vi "DROPBEAR_Model_Updating_Store_Statisitics.vi"(8 "error in (no error)":errorcluster, 11 "DROPBEAR_Model_Updating in":refnum<class "DROPBEAR_Model_Updating.lvclass">) -> (0 "error out":errorcluster, 3 "DROPBEAR_Model_Updating out":refnum<class "DROPBEAR_Model_Updating.lvclass">)   [LabVIEW 2021, in "DROPBEAR_Model_Updating.lvclass"]
uses:
  DROPBEAR_Model_Updating.lvclass
  Online_Statistic/Online_Statistic.lvclass
  Moving_Statistic/Moving_Statistic.lvclass
  Data_Array/Data_Array.lvclass
  DROPBEAR_Model_Updating.lvclass/DROPBEAR_Model_Updating.ctl
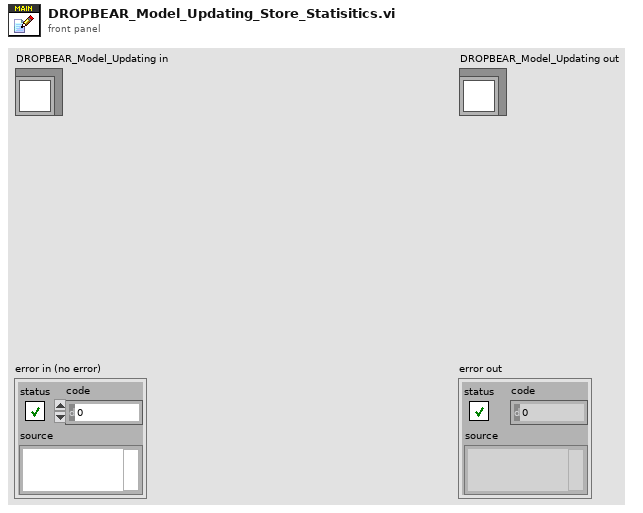
[diagram p1: front panel]
types:
  T1 = cluster{"Data Acquistion Time Cost":refnum<class "Online_Statistic.lvclass">, "FFT Time Cost":refnum<class "Online_Statistic.lvclass">, "Sample Location Time Cost":refnum<class "Online_Statistic.lvclass">, "FEA Time Cost":refnum<class "Online_Statistic.lvclass">, "Frequency Tracking Time Cost":refnum<class "Online_Statistic.lvclass">, "State Tracking Time Cost":refnum<class "Online_Statistic.lvclass">, "Online Cycle Time Cost":refnum<class "Online_Statistic.lvclass">}
  T2 = cluster{"Time Cycle Start":u32, "Time Data Acquire":u32, "Time FFT":u32, "Time KF FFT":u32, "Time Sample":u32, "Time FEA":u32, "Time KF FEA":u32, "Time Cycle End":u32}
  T3 = cluster{"Number_of_samples":i32, "Max":dbl, "Min":dbl, "Cumulative_mean":dbl, "Cumulative_mean_square ":dbl, "Cumulative_variance":dbl}
  T4 = cluster{"Displacement Measured Meters":refnum<class "Moving_Statistic.lvclass">, "Displacement Estimate Meters":refnum<class "Moving_Statistic.lvclass">, "Frequency Measured":refnum<class "Moving_Statistic.lvclass">, "Frequency at Estimate":refnum<class "Moving_Statistic.lvclass">}
  T5 = cluster{"Position Measured Meters":dbl, "Position Measured Nodal":i32, "Position Estimated Meters":dbl, "Position Estimated Nodal":i32, "Frequency Estimated KF":dbl, "Frequency Measured FFT":dbl, "Position Estimated Meters KF":dbl, "Position Estimated Nodal KF":i32, "Mean Cycle time":dbl}
  T6 = cluster{"Modeling Parameters input controls":cluster{"beam_length":dbl, "youngs_modulus":dbl, "torsion_spring":dbl, "beam_height":dbl, "beam_width":dbl, "beam_density":dbl, "number_of_FEA_nodes":i32, "accelerometer_mass":dbl}, "Mockbear input controls":cluster{"Dataset":string, "Resample Method":enum16{"Recorded", "Auto Resample", "Custom Resample"}}, "Simulation Parameters input controls":cluster{"Eigensolver ":enum16{"LabVIEW Cholesky", "LabVIEW General", "LabVIEW Inverse", "LEMP"}, "Models Forcasted":i32, "Max Roller Velocity":dbl, "Max Roller Position Percent":dbl, "Min Roller Position Percent":dbl}, "Program Controls":cluster{"Frequency KF":bool, "Pinned State KF":bool, "FFT Bounding":bool, "Filter Constants Frequency":cluster{"Measurement Variance":dbl, "State Variance":dbl, "Threshold":dbl}, "Filter Constants Position":cluster{"Measurement Variance":dbl, "State Variance":dbl, "Threshold":dbl}, "Moving Window Size":dbl}}
  T7 = cluster{"Frequency KF":bool, "Pinned State KF":bool, "FFT Bounding":bool, "Filter Constants Frequency":cluster{"Measurement Variance":dbl, "State Variance":dbl, "Threshold":dbl}, "Filter Constants Position":cluster{"Measurement Variance":dbl, "State Variance":dbl, "Threshold":dbl}, "Moving Window Size":dbl}
  T8 = cluster{"Displacement Measured Nodal ":refnum<class "Data_Array.lvclass">, "Displacement Measured Meters":refnum<class "Data_Array.lvclass">, "Displacement Estimate Nodal":refnum<class "Data_Array.lvclass">, "Displacement Estimate Meters":refnum<class "Data_Array.lvclass">, "Frequency Measured":refnum<class "Data_Array.lvclass">, "Frequency at Estimate":refnum<class "Data_Array.lvclass">}
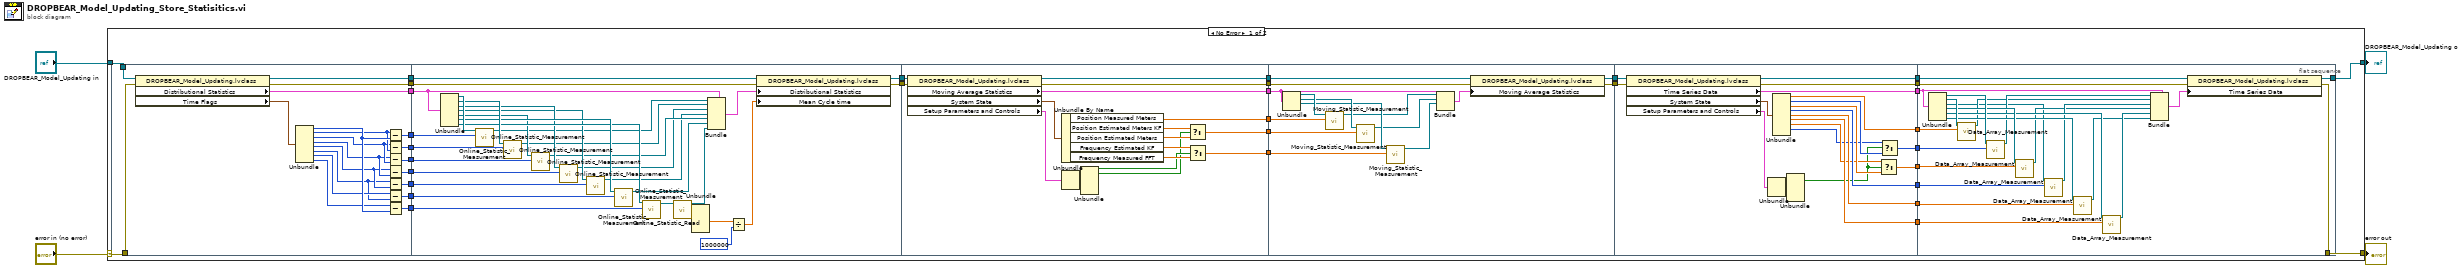
[diagram p0: block diagram]
diagram:
  n1 = case shown="No Error" "error in (no error)" {
    selector: "error in (no error)" -> [w5 w167]
    tunnel: [w6 w167] -> w3
    tunnel: [w7 w166] -> w1
    tunnel: "DROPBEAR_Model_Updating in" -> [w37 w166]
    frame No Error {
      n2 = flat-sequence {
        tunnel: w37 -> [w58]
        tunnel: [w53] -> w36
        tunnel: [w52] -> w35
        tunnel: [w51] -> w34
        tunnel: [w50] -> w33
        tunnel: [w49] -> w32
        tunnel: [w48] -> w31
        tunnel: [w47] -> w30
        tunnel: [w46] -> w29
        tunnel: [w40] -> w28
        tunnel: [w39] -> w26
        tunnel: w5 -> [w38]
        tunnel: w36 -> [w77]
        tunnel: w35 -> [w90]
        tunnel: w34 -> [w89]
        tunnel: w33 -> [w88]
        tunnel: w32 -> [w87]
        tunnel: w31 -> [w86]
        tunnel: w30 -> [w85]
        tunnel: w29 -> [w64]
        tunnel: w28 -> [w69]
        tunnel: [w67] -> w27
        tunnel: w26 -> [w66]
        tunnel: [w65] -> w25
        tunnel: w27 -> [w107]
        tunnel: w25 -> [w106]
        tunnel: [w105] -> w24
        tunnel: [w103] -> w23
        tunnel: [w94] -> w22
        tunnel: [w93] -> w21
        tunnel: [w92] -> w20
        tunnel: [w91] -> w19
        tunnel: w24 -> [w116]
        tunnel: w23 -> [w119]
        tunnel: w22 -> [w118]
        tunnel: w21 -> [w117]
        tunnel: w20 -> [w112]
        tunnel: w19 -> [w111]
        tunnel: [w109] -> w18
        tunnel: [w108] -> w17
        tunnel: w18 -> [w141]
        tunnel: w17 -> [w140]
        tunnel: [w138] -> w16
        tunnel: [w137] -> w15
        tunnel: [w128] -> w14
        tunnel: [w131] -> w13
        tunnel: [w136] -> w12
        tunnel: [w135] -> w11
        tunnel: [w134] -> w10
        tunnel: [w125] -> w9
        tunnel: [w124] -> w8
        tunnel: w16 -> [w165]
        tunnel: w15 -> [w164]
        tunnel: w14 -> [w161]
        tunnel: w13 -> [w159]
        tunnel: w12 -> [w158]
        tunnel: w11 -> [w157]
        tunnel: w10 -> [w156]
        tunnel: w9 -> [w153]
        tunnel: w8 -> [w152]
        tunnel: [w143] -> w7
        tunnel: [w142] -> w6
        frame #0 {
          n3 = property class="DROPBEAR_Model_Updating.lvclass"(reference=w58, error in=w38) -> (reference out=w40:refnum<class "DROPBEAR_Model_Updating.lvclass">, error out=w39:errorcluster, "Distributional Statistics"=w53:T1, "Time Flags"=w57:T2)
          n4 = Unbundle(w57) -> ("Time Cycle Start"=w56:u32, "Time Data Acquire"=w45:u32, "Time FFT"=w44:u32, "Time KF FFT"=w43:u32, "Time Sample"=w42:u32, "Time FEA"=w41:u32, "Time KF FEA"=w55:u32, "Time Cycle End"=w54:u32)
          n5 = Subtract(x=w45, y=w56) -> (x-y=w52:u32)
          n6 = Subtract(x=w44, y=w45) -> (x-y=w51:u32)
          n7 = Subtract(x=w43, y=w44) -> (x-y=w50:u32)
          n8 = Subtract(x=w42, y=w43) -> (x-y=w49:u32)
          n9 = Subtract(x=w41, y=w42) -> (x-y=w48:u32)
          n10 = Subtract(x=w55, y=w41) -> (x-y=w47:u32)
          n11 = Subtract(x=w54, y=w56) -> (x-y=w46:u32)
        }
        frame #1 {
          n12 = Unbundle(w77) -> ("Data Acquistion Time Cost"=w84:refnum<class "Online_Statistic.lvclass">, "FFT Time Cost"=w83:refnum<class "Online_Statistic.lvclass">, "Sample Location Time Cost"=w79:refnum<class "Online_Statistic.lvclass">, "FEA Time Cost"=w78:refnum<class "Online_Statistic.lvclass">, "Frequency Tracking Time Cost"=w80:refnum<class "Online_Statistic.lvclass">, "State Tracking Time Cost"=w82:refnum<class "Online_Statistic.lvclass">, "Online Cycle Time Cost"=w81:refnum<class "Online_Statistic.lvclass">)
          n13 = call-dynamic "Online_Statistic_Measurement.vi"("New_Measurement"=w90, "Online_Statistic in"=w84) -> ("Online_Statistic out"=w76:refnum<class "Online_Statistic.lvclass">)  [unwired: 8 in, 1 out]
          n14 = call-dynamic "Online_Statistic_Measurement.vi"("New_Measurement"=w89, "Online_Statistic in"=w83) -> ("Online_Statistic out"=w75:refnum<class "Online_Statistic.lvclass">)  [unwired: 8 in, 1 out]
          n15 = call-dynamic "Online_Statistic_Measurement.vi"("New_Measurement"=w88, "Online_Statistic in"=w80) -> ("Online_Statistic out"=w74:refnum<class "Online_Statistic.lvclass">)  [unwired: 8 in, 1 out]
          n16 = call-dynamic "Online_Statistic_Measurement.vi"("New_Measurement"=w87, "Online_Statistic in"=w79) -> ("Online_Statistic out"=w73:refnum<class "Online_Statistic.lvclass">)  [unwired: 8 in, 1 out]
          n17 = call-dynamic "Online_Statistic_Measurement.vi"("New_Measurement"=w86, "Online_Statistic in"=w78) -> ("Online_Statistic out"=w72:refnum<class "Online_Statistic.lvclass">)  [unwired: 8 in, 1 out]
          n18 = call-dynamic "Online_Statistic_Measurement.vi"("New_Measurement"=w85, "Online_Statistic in"=w82) -> ("Online_Statistic out"=w71:refnum<class "Online_Statistic.lvclass">)  [unwired: 8 in, 1 out]
          n19 = call-dynamic "Online_Statistic_Measurement.vi"("New_Measurement"=w64, "Online_Statistic in"=w81) -> ("Online_Statistic out"=w70:refnum<class "Online_Statistic.lvclass">)  [unwired: 8 in, 1 out]
          n20 = call-dynamic "Online_Statistic_Read.vi"("Online_Statistic in"=w70) -> ("stats_private"=w60:T3, "Online_Statistic out"=w61:refnum<class "Online_Statistic.lvclass">)  [unwired: 8 in, 1 out]
          n21 = Unbundle(w60) -> ("Cumulative_mean"=w59:dbl)  [unwired: 5 out]
          n22 = Bundle(cluster=w77, "Data Acquistion Time Cost"=w76, "FFT Time Cost"=w75, "Sample Location Time Cost"=w73, "FEA Time Cost"=w72, "Frequency Tracking Time Cost"=w74, "State Tracking Time Cost"=w71, "Online Cycle Time Cost"=w61) -> (w68:T1)
          n23 = Divide(x=w59, y=u32 1000000) -> (x/y=w62:dbl)
          n24 = property class="DROPBEAR_Model_Updating.lvclass"(reference=w69, error in=w66, "Distributional Statistics"=w68, "Mean Cycle time"=w62) -> (reference out=w67:refnum<class "DROPBEAR_Model_Updating.lvclass">, error out=w65:errorcluster)
        }
        frame #2 {
          n25 = property class="DROPBEAR_Model_Updating.lvclass"(reference=w107, error in=w106) -> (reference out=w92:refnum<class "DROPBEAR_Model_Updating.lvclass">, error out=w91:errorcluster, "Moving Average Statistics"=w105:T4, "System State"=w104:T5, "Setup Parameters and Controls"=w102:T6)
          n26 = Unbundle By Name(w104) -> ("Position Measured Meters"=w103:dbl, "Position Estimated Meters KF"=w100:dbl, "Position Estimated Meters"=w99:dbl, "Frequency Estimated KF"=w98:dbl, "Frequency Measured FFT"=w97:dbl)
          n27 = Unbundle(w102) -> ("Program Controls"=w101:T7)  [unwired: 3 out]
          n28 = Unbundle(w101) -> ("Frequency KF"=w96:bool, "Pinned State KF"=w95:bool)  [unwired: 4 out]
          n29 = Select(t=w100, s=w95, f=w99) -> (s? t:f=w94:dbl)
          n30 = Select(t=w98, s=w96, f=w97) -> (s? t:f=w93:dbl)
        }
        frame #3 {
          n31 = Unbundle(w116) -> ("Displacement Measured Meters"=w122:refnum<class "Moving_Statistic.lvclass">, "Displacement Estimate Meters"=w121:refnum<class "Moving_Statistic.lvclass">, "Frequency Measured"=w120:refnum<class "Moving_Statistic.lvclass">)  [unwired: 1 out]
          n32 = call-dynamic "Moving_Statistic_Measurement.vi"("New_Measurement"=w119, "Moving_Mean in"=w122) -> ("Moving_Mean out"=w115:refnum<class "Moving_Statistic.lvclass">)  [unwired: 8 in, 1 out]
          n33 = call-dynamic "Moving_Statistic_Measurement.vi"("New_Measurement"=w118, "Moving_Mean in"=w121) -> ("Moving_Mean out"=w114:refnum<class "Moving_Statistic.lvclass">)  [unwired: 8 in, 1 out]
          n34 = call-dynamic "Moving_Statistic_Measurement.vi"("New_Measurement"=w117, "Moving_Mean in"=w120) -> ("Moving_Mean out"=w113:refnum<class "Moving_Statistic.lvclass">)  [unwired: 8 in, 1 out]
          n35 = Bundle(cluster=w116, "Displacement Measured Meters"=w115, "Displacement Estimate Meters"=w114, "Frequency Measured"=w113) -> (w110:T4)  [unwired: 1 in]
          n36 = property class="DROPBEAR_Model_Updating.lvclass"(reference=w112, error in=w111, "Moving Average Statistics"=w110) -> (reference out=w109:refnum<class "DROPBEAR_Model_Updating.lvclass">, error out=w108:errorcluster)
        }
        frame #4 {
          n37 = property class="DROPBEAR_Model_Updating.lvclass"(reference=w141, error in=w140) -> (reference out=w125:refnum<class "DROPBEAR_Model_Updating.lvclass">, error out=w124:errorcluster, "Time Series Data"=w138:T8, "System State"=w139:T5, "Setup Parameters and Controls"=w132:T6)
          n38 = Unbundle(w132) -> ("Program Controls"=w133:T7)  [unwired: 3 out]
          n39 = Unbundle(w139) -> ("Position Measured Meters"=w137:dbl, "Position Measured Nodal"=w127:i32, "Position Estimated Meters"=w130:dbl, "Position Estimated Nodal"=w136:i32, "Frequency Estimated KF"=w135:dbl, "Frequency Measured FFT"=w134:dbl, "Position Estimated Meters KF"=w129:dbl, "Position Estimated Nodal KF"=w126:i32)  [unwired: 1 out]
          n40 = Unbundle(w133) -> ("Pinned State KF"=w123:bool)  [unwired: 5 out]
          n41 = Select(t=w129, s=w123, f=w130) -> (s? t:f=w131:dbl)
          n42 = Select(t=w126, s=w123, f=w127) -> (s? t:f=w128:i32)
        }
        frame #5 {
          n43 = Unbundle(w165) -> ("Displacement Measured Nodal"=w162:refnum<class "Data_Array.lvclass">, "Displacement Measured Meters"=w163:refnum<class "Data_Array.lvclass">, "Displacement Estimate Nodal"=w144:refnum<class "Data_Array.lvclass">, "Displacement Estimate Meters"=w160:refnum<class "Data_Array.lvclass">, "Frequency Measured"=w155:refnum<class "Data_Array.lvclass">, "Frequency at Estimate"=w154:refnum<class "Data_Array.lvclass">)
          n44 = call-dynamic "Data_Array_Measurement.vi"("Measurement"=w164, "Data_Array in"=w163) -> ("Data_Array out"=w145:refnum<class "Data_Array.lvclass">)  [unwired: 8 in, 1 out]
          n45 = call-dynamic "Data_Array_Measurement.vi"("Measurement"=w161, "Data_Array in"=w162) -> ("Data_Array out"=w146:refnum<class "Data_Array.lvclass">)  [unwired: 8 in, 1 out]
          n46 = call-dynamic "Data_Array_Measurement.vi"("Measurement"=w159, "Data_Array in"=w160) -> ("Data_Array out"=w147:refnum<class "Data_Array.lvclass">)  [unwired: 8 in, 1 out]
          n47 = call-dynamic "Data_Array_Measurement.vi"("Measurement"=w158, "Data_Array in"=w144) -> ("Data_Array out"=w148:refnum<class "Data_Array.lvclass">)  [unwired: 8 in, 1 out]
          n48 = call-dynamic "Data_Array_Measurement.vi"("Measurement"=w157, "Data_Array in"=w154) -> ("Data_Array out"=w149:refnum<class "Data_Array.lvclass">)  [unwired: 8 in, 1 out]
          n49 = call-dynamic "Data_Array_Measurement.vi"("Measurement"=w156, "Data_Array in"=w155) -> ("Data_Array out"=w150:refnum<class "Data_Array.lvclass">)  [unwired: 8 in, 1 out]
          n50 = Bundle(cluster=w165, "Displacement Measured Nodal"=w146, "Displacement Measured Meters"=w145, "Displacement Estimate Nodal"=w148, "Displacement Estimate Meters"=w147, "Frequency Measured"=w150, "Frequency at Estimate"=w149) -> (w151:T8)
          n51 = property class="DROPBEAR_Model_Updating.lvclass"(reference=w153, error in=w152, "Time Series Data"=w151) -> (reference out=w143:refnum<class "DROPBEAR_Model_Updating.lvclass">, error out=w142:errorcluster)
        }
      }
    }
    frame Error {
    }
  }
  "error out" <- w3
  "DROPBEAR_Model_Updating out" <- w1
